vi "ExSubCreateFileStrip.vi"(2 "error in (no error)":errorcluster, 3 "File and Display Name":string, 4 "Pulser Handle":u32, 5 "Camera Handle":u32) -> (0 "error out":errorcluster, 1 "Handles Out":T1)   [LabVIEW 2010]
panel:
  # "ExSubCreateFileStrip:\nThis Sub-VI creates a file and opens it"
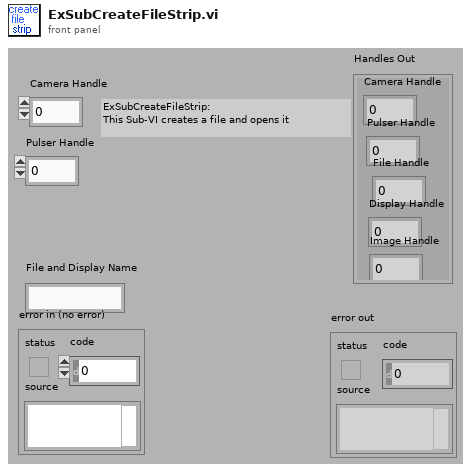
[diagram p1: front panel]
types:
  T1 = cluster{"Camera Handle":u32, "Pulser Handle":u32, "File Handle":u32, "Display Handle":u32, "Image Handle":u32}
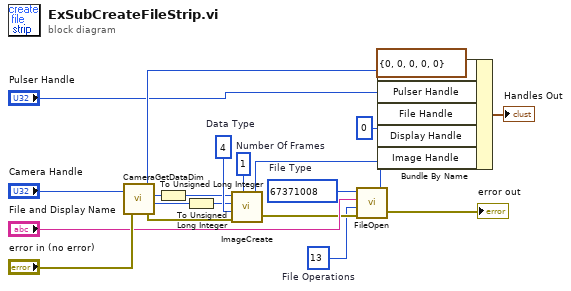
[diagram p0: block diagram]
diagram:
  w9 = 13  # File Operations
  w10 = 67371008  # File Type
  w11 = u32 4  # Data Type
  w12 = u32 1  # Number Of Frames
  n1 = call <userlib>:"CameraGetDataDim.vi"("Camera Handle"="Camera Handle", "error in"="error in (no error)") -> ("Camera Handle"=w8:u32, "Xdim"=w19:u32, "Ydim"=w20:u32, "error out"=w21:errorcluster)
  n2 = To Unsigned Long Integer(number=w19) -> (unsigned 32bit integer=w3:u32)
  n3 = To Unsigned Long Integer(number=w20) -> (unsigned 32bit integer=w2:u32)
  n4 = call <userlib>:"ImageCreate.vi"("X dimension"=w3, "Y dimension"=w2, "Data Type"=w11, "error in"=w21, "Number Of Frames"=w12) -> ("Image Handle"=w6:u32, "error out"=w13:errorcluster)
  n5 = call <userlib>:"FileOpen.vi"("error in"=w13, "File Operations"=w9, "FileName"="File and Display Name", "File Type"=w10) -> ("error out"=→"error out":errorcluster, "File Handle"=w5:u32)
  n6 = Bundle By Name(cluster=T1 {"Camera Handle"=0, "Pulser Handle"=0, "File Handle"=0, "Display Handle"=0, "Image Handle"=0} ("Handles Out"), "Camera Handle"=w8, "Pulser Handle"="Pulser Handle", "File Handle"=w5, "Display Handle"=u32 0, "Image Handle"=w6) -> (→"Handles Out":T1)
